vi "Test Stub.vi"(11 "Test Case In":refnum<class "Tests Event MessengerM.lvclass">) -> (0 "error out":errorcluster, 3 "Test Case Out":refnum<class "Tests Event MessengerM.lvclass">)   [LabVIEW 2020, in "Tests Event MessengerM.lvclass"]
uses:
  Tests Event MessengerM.lvclass
  C:/Program Files/National Instruments/LabVIEW 2020/vi.lib/Astemes/LUnit/Test Case.lvclass
  <vilib>/Astemes/LUnit/Test Case.lvclass/Test Case.ctl
  <vilib>/Astemes/LUnit/Core/LUnit Test Case/Private/Append Fail Result.vi
  <vilib>/Astemes/LUnit/Core/LUnit Test Case/Private/Append Pass Result.vi
  <vilib>/Astemes/LUnit/Core/LUnit Test Case/Private/Run In UI.vi
  <vilib>/Utility/error.llb/Clear Errors.vi
  <extravilib>/ChannelInstances/Event MessengerM-i32/Instantiate.vi
  <extravilib>/ChannelInstances/Event MessengerM-i32/))Channel.vi
  Tests Event MessengerM.lvclass/Tests Event MessengerM.ctl
  <vilib>/Astemes/LUnit/Test Case.lvclass
  <extravilib>/ChannelInstances/Event MessengerM-i32.lvlib
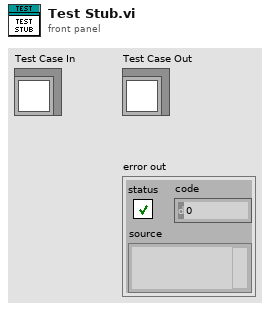
[diagram p1: front panel]
types:
  T1 = typedef "Event MessengerM-i32.lvlib/))Channel.ctl" = refnum<queue>
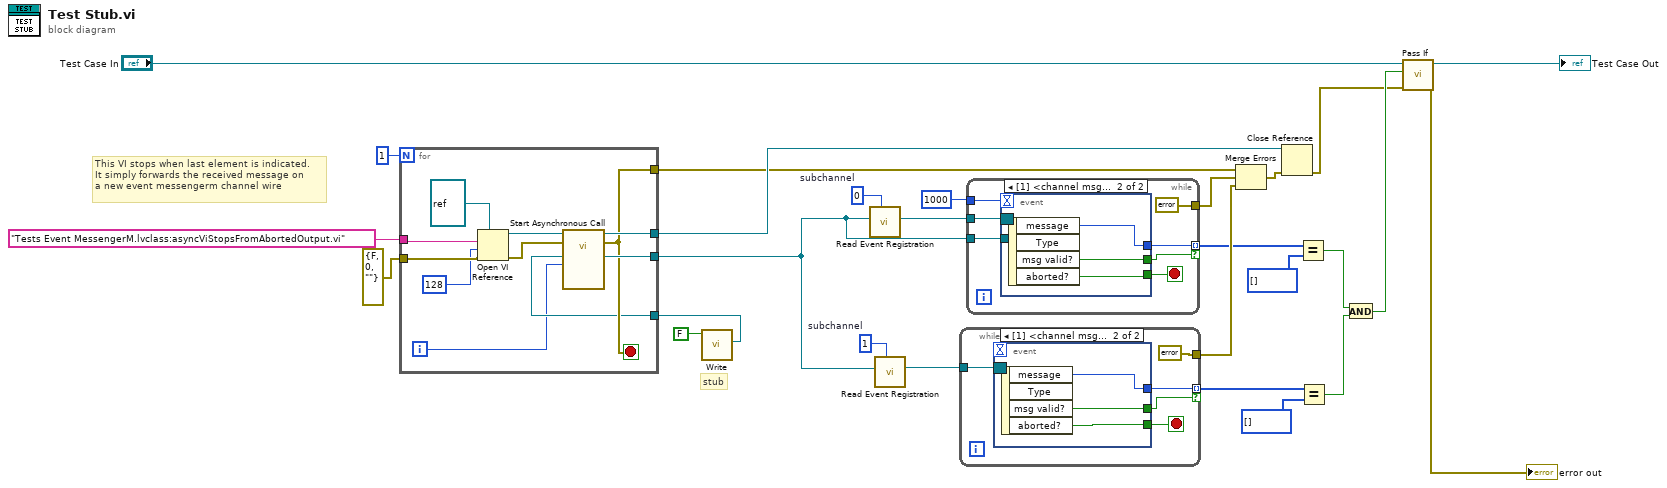
[diagram p0: block diagram]
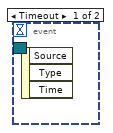
[diagram p2: hidden frame]
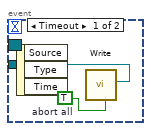
[diagram p3: hidden frame]
diagram:
  w2 = 1  # subchannel
  w5 = 0  # subchannel
  # "stub"
  # "This VI stops when last element is indicated.\nIt simply forwards the received message on\na new event messengerm channel wire"
  n1 = call <extravilib>:"Write.vi"("element valid? (T)"=FALSE) -> ("channel"=w7:T1)  [unwired: 9 in, 1 out]
  n2 = for {
    N: 1 -> [_]
    tunnel: "Tests Event MessengerM.lvclass:asyncViStopsFromAbortedOutput.vi" -> [w38]
    tunnel: errorcluster {"status"=FALSE, "code"=0, "source"=""} ("error constant") -> [w34]
    tunnel: [w33] -> w3
    tunnel: [w32] -> w17
    tunnel: [w30] -> w15
    tunnel: w7 -> [w29]
    i -> [w28]
    stop <- w30 stop-if-true
    n3 = Open VI Reference(type specifier VI Refnum (for type only)=refnum<vi> refnum, vi path=w38, options=128, error in (no error)=w34) -> (vi reference=w36:refnum<vi>, error out=w35:errorcluster)  [unwired: 2 in]
    n4 = call-by-ref "Start Asynchronous Call"(reference=w36, error in=w35, "subchannel (0)"=w28, "channel"=w29) -> (reference out=w32:refnum<vi>, error out=w30:errorcluster, "other channel"=w33:T1)  [unwired: 9 in]
  }
  n5 = call <extravilib>:"Read Event Registration.vi"("subchannel (0)"=w5, "channel"=w3) -> ("event registration refnum"=w4:refnum<event-registration>)  [unwired: 9 in]
  n6 = call <extravilib>:"Read Event Registration.vi"("subchannel (0)"=w2, "channel"=w3) -> ("event registration refnum"=w1:refnum<event-registration>)  [unwired: 9 in]
  n7 = while {
    tunnel: w1 -> [w43]
    tunnel: [errorcluster {"status"=FALSE, "code"=0, "source"=""} ("error constant")] -> w20
    tunnel: [w41] -> w13 mode=indexing if=w39
    stop <- w40 stop-if-true
    n8 = event shown="[1] <channel msg>: User Event" {
      selector: w43 -> [_ _]
      dyn-events: _ -> [_ _]
      timeout: _ -> [_ _]
      tunnel: [_ w46] -> w41
      tunnel: [_ w45] -> w40
      tunnel: [_ w44] -> w39
      event Timeout {
        n9 = event-data() -> ()  [unwired: 1 in, 3 out]
      }
      event User Event {
        n10 = event-data() -> ("message"=w46:i32, "msg valid?"=w44:bool, "aborted?"=w45:bool)  [unwired: 1 in, 1 out]
      }
    }
  }
  n11 = while {
    tunnel: w4 -> [w53]
    tunnel: [errorcluster {"status"=FALSE, "code"=0, "source"=""} ("error constant")] -> w19
    tunnel: [w51] -> w14 mode=indexing if=w47
    tunnel: 1000 -> [w49]
    tunnel: w3 -> [w48]
    stop <- w50 stop-if-true
    n12 = event shown="[1] <channel msg>: User Event" {
      selector: w53 -> [_ _]
      dyn-events: _ -> [_ _]
      timeout: w49 -> [_ _]
      tunnel: [_ w58] -> w51
      tunnel: [_ w57] -> w50
      tunnel: [w55 _] -> w48
      tunnel: [_ w56] -> w47
      event Timeout {
        w54 = TRUE  # abort all
        n13 = event-data() -> ()  [unwired: 1 in, 3 out]
        n14 = call <extravilib>:"Write.vi"("abort all (F)"=w54) -> ("channel"=w55:T1)  [unwired: 9 in, 1 out]
      }
      event User Event {
        n15 = event-data() -> ("message"=w58:i32, "msg valid?"=w56:bool, "aborted?"=w57:bool)  [unwired: 1 in, 1 out]
      }
    }
  }
  n16 = Merge Errors(w15, w19, w20) -> (w18:errorcluster)
  n17 = Close Reference(reference=w17, error in (no error)=w18) -> (error out=w16:errorcluster)
  n18 = Equal?(x=w14, y=i32[] []) -> (x = y?=w10:bool)
  n19 = Equal?(x=w13, y=i32[] []) -> (x = y?=w9:bool)
  n20 = And(x=w10, y=w9) -> (x .and. y?=w24:bool)
  n21 = call <vilib>:"Pass If.vi"("error in (no error)"=w16, "Pass?"=w24, "LUnit Test Case In"="Test Case In") -> ("error out"=→"error out":errorcluster, "LUnit Test Case Out"=→"Test Case Out":refnum<class "Tests Event MessengerM.lvclass">)  [unwired: 7 in]
